vi "S11_calculations.vi"(9 "S11_Imag":dbl[](array[numeric]), 10 "S11_Real":dbl[](array[numeric]), 11 "Frequency":dbl[](array[numeric])) -> (1 "Complex":T2, 2 "Calc":T1, 3 "Raw":T3)   [LabVIEW 2020]
panel:
  out "r":dbl[](array[numeric])
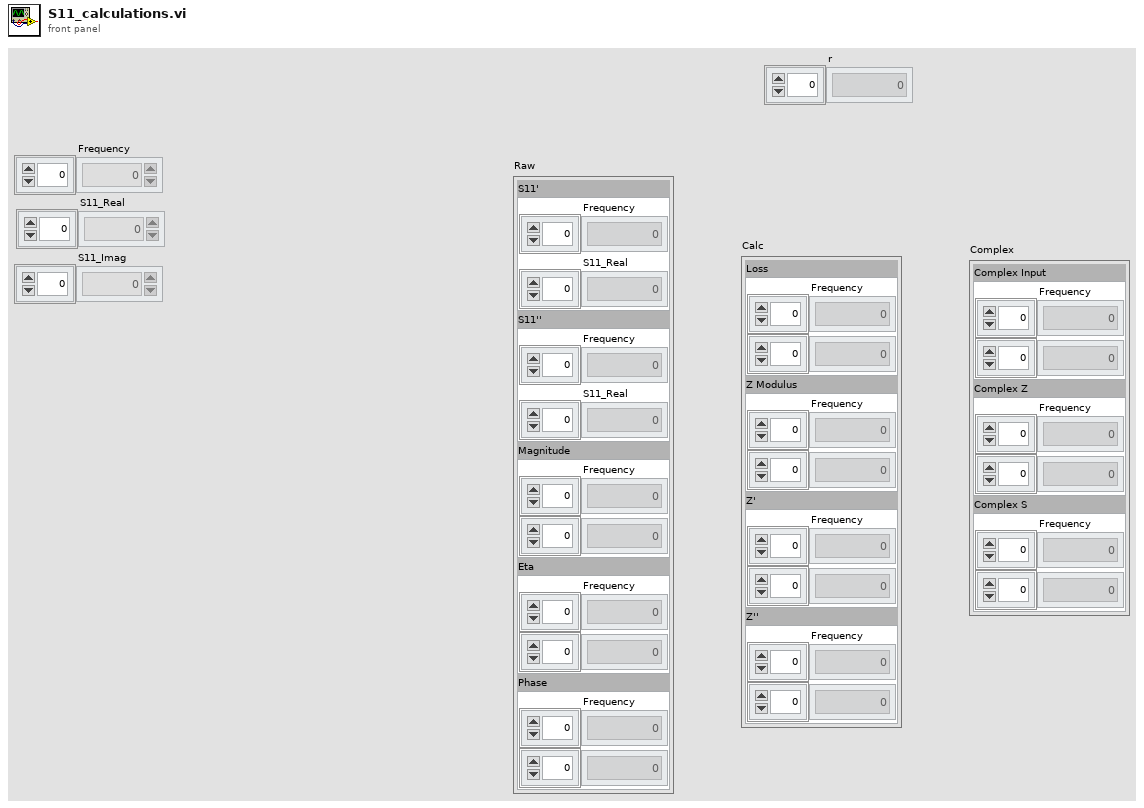
[diagram p1: front panel]
types:
  T1 = cluster{"Loss":cluster{"Frequency":dbl[], "Array":dbl[]}, "Z Modulus":cluster{"Frequency":dbl[], "Array":dbl[]}, "Z'":cluster{"Frequency":dbl[], "Array":dbl[]}, "Z''":cluster{"Frequency":dbl[], "Array":dbl[]}}
  T2 = cluster{"Complex Input":cluster{"Frequency":dbl[], "Array":cdb[]}, "Complex Z":cluster{"Frequency":dbl[], "Array":cdb[]}, "Complex S":cluster{"Frequency":dbl[], "Array":cdb[]}}
  T3 = cluster{"S11'":cluster{"Frequency":dbl[], "S11_Real":dbl[]}, "S11''":cluster{"Frequency":dbl[], "S11_Real":dbl[]}, "Magnitude":cluster{"Frequency":dbl[], "Array":dbl[]}, "Eta":cluster{"Frequency":dbl[], "Array":dbl[]}, "Phase":cluster{"Frequency":dbl[], "Array":dbl[]}}
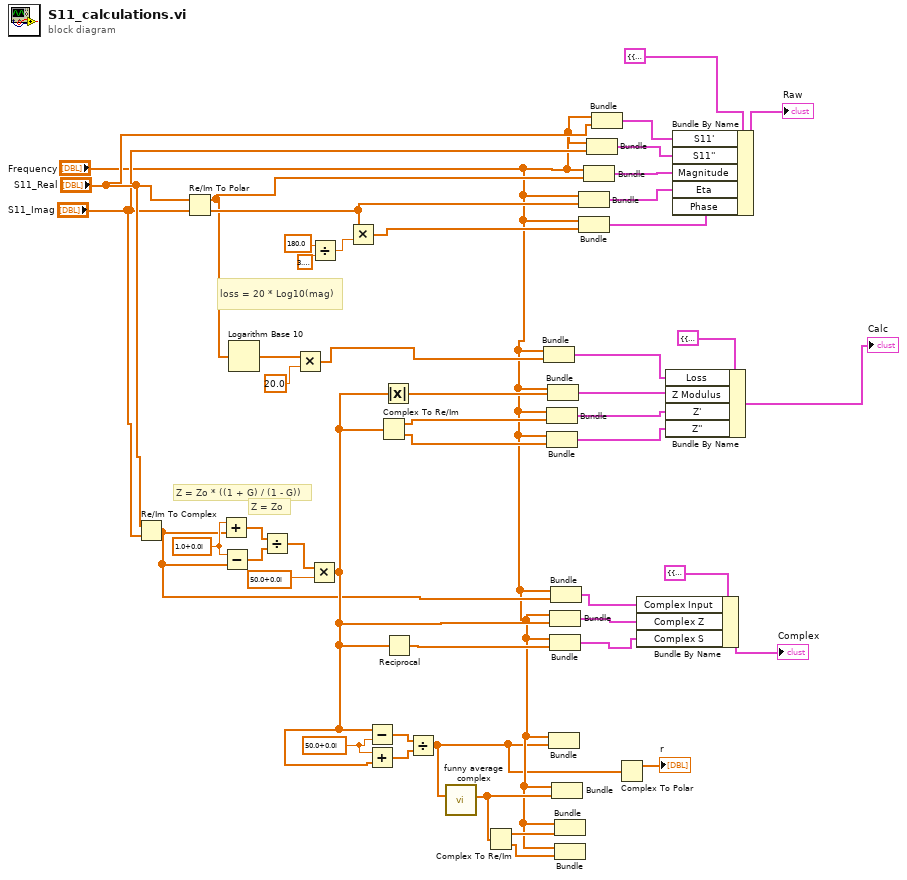
[diagram p0: block diagram]
diagram:
  w30 = cdb 50.0+0.0i ("y")
  w44 = cdb 1.0+0.0i ("x")
  # "Z = Zo"
  # "Z = Zo * ((1 + G) / (1 - G))"
  # "loss = 20 * Log10(mag)"
  n1 = Re/Im To Complex(1:"S11_Imag", 2:"S11_Real") -> (0:w24:cdb[])
  n2 = Re/Im To Polar(2:"S11_Imag", 3:"S11_Real") -> (0:w38:dbl[], 1:w29:dbl[])
  n3 = Add(x=w44, y=w24) -> (x+y=w43:cdb[])
  n4 = Subtract(x=w44, y=w24) -> (x-y=w42:cdb[])
  n5 = Logarithm Base 10(1:w29) -> (0:w46:dbl[])
  n6 = Divide(x=w43, y=w42) -> (x/y=w41:cdb[])
  n7 = Multiply(x=w46, y=20.0) -> (x*y=w36:dbl[])
  n8 = Multiply(x=w41, y=cdb 50.0+0.0i) -> (x*y=w25:cdb[])
  n9 = Divide(x=180.0, y=3.141592653589793) -> (x/y=w47:dbl)
  n10 = Multiply(x=w38, y=w47) -> (x*y=w37:dbl[])
  n11 = Subtract(x=w25, y=w30) -> (x-y=w32:cdb[])
  n12 = Add(x=w30, y=w25) -> (x+y=w31:cdb[])
  n13 = Complex To Re/Im(x + iy=w25) -> (x=w34:dbl[], y=w33:dbl[])
  n14 = Absolute Value(x=w25) -> (abs(x)=w35:dbl[])
  n15 = Reciprocal(x=w25) -> (1/x=w39:cdb[])
  n16 = Divide(x=w32, y=w31) -> (x/y=w2:cdb[])
  n17 = call "funny average complex.vi"("in"=w2) -> ("Out"=w28:cdb[])  [unwired: 10 in]
  n18 = Complex To Re/Im(x + iy=w28) -> (x=w27:dbl[], y=w26:dbl[])
  n19 = Bundle("Frequency"="Frequency", w36) -> (w12:cluster{"Frequency":dbl[], dbl[]})  [unwired: 1 in]
  n20 = Bundle("Frequency"="Frequency", w34) -> (w10:cluster{"Frequency":dbl[], dbl[]})  [unwired: 1 in]
  n21 = Bundle("Frequency"="Frequency", w33) -> (w9:cluster{"Frequency":dbl[], dbl[]})  [unwired: 1 in]
  n22 = Bundle("Frequency"="Frequency", w35) -> (w11:cluster{"Frequency":dbl[], dbl[]})  [unwired: 1 in]
  n23 = Bundle("Frequency"="Frequency", w2) -> ()  [unwired: 1 in, 1 out]
  n24 = Bundle("Frequency"="Frequency", w25) -> (w5:cluster{"Frequency":dbl[], cdb[]})  [unwired: 1 in]
  n25 = Bundle("Frequency"="Frequency", w39) -> (w4:cluster{"Frequency":dbl[], cdb[]})  [unwired: 1 in]
  n26 = Bundle("Frequency"="Frequency", w24) -> (w6:cluster{"Frequency":dbl[], cdb[]})  [unwired: 1 in]
  n27 = Bundle("Frequency"="Frequency", "Out"=w28) -> ()  [unwired: 1 in, 1 out]
  n28 = Bundle("Frequency"="Frequency", w27) -> ()  [unwired: 1 in, 1 out]
  n29 = Bundle("Frequency"="Frequency", w26) -> ()  [unwired: 1 in, 1 out]
  n30 = Bundle("Frequency"="Frequency", w38) -> (w16:cluster{"Frequency":dbl[], dbl[]})  [unwired: 1 in]
  n31 = Bundle("Frequency"="Frequency", w37) -> (w15:cluster{"Frequency":dbl[], dbl[]})  [unwired: 1 in]
  n32 = Bundle("Frequency"="Frequency", w29) -> (w17:cluster{"Frequency":dbl[], dbl[]})  [unwired: 1 in]
  n33 = Bundle("Frequency"="Frequency", "S11_Imag"="S11_Imag") -> (w18:cluster{"Frequency":dbl[], "S11_Imag":dbl[]})  [unwired: 1 in]
  n34 = Bundle("Frequency"="Frequency", "S11_Real"="S11_Real") -> (w19:cluster{"Frequency":dbl[], "S11_Real":dbl[]})  [unwired: 1 in]
  n35 = Complex To Polar(r * e^(i*theta)=w2) -> (r=→"r":dbl[])  [unwired: 1 out]
  n36 = Bundle By Name(cluster=T2 {"Complex Input"={"Frequency"=[], "Array"=[]}, "Complex Z"={"Frequency"=[], "Array"=[]}, "Complex S"={"Frequency"=[], "Array"=[]}} ("Complex"), "Complex Input"=w6, "Complex Z"=w5, "Complex S"=w4) -> (→"Complex":T2)
  n37 = Bundle By Name(cluster=T1 {"Loss"={"Frequency"=[], "Array"=[]}, "Z Modulus"={"Frequency"=[], "Array"=[]}, "Z'"={"Frequency"=[], "Array"=[]}, "Z''"={"Frequency"=[], "Array"=[]}} ("Calc"), "Loss"=w12, "Z Modulus"=w11, "Z'"=w10, "Z''"=w9) -> (→"Calc":T1)
  n38 = Bundle By Name(cluster=T3 {"S11'"={"Frequency"=[], "S11_Real"=[]}, "S11''"={"Frequency"=[], "S11_Real"=[]}, "Magnitude"={"Frequency"=[], "Array"=[]}, "Eta"={"Frequency"=[], "Array"=[]}, "Phase"={"Frequency"=[], "Array"=[]}} ("Raw"), "S11'"=w19, "S11''"=w18, "Magnitude"=w17, "Eta"=w16, "Phase"=w15) -> (→"Raw":T3)
